vi "Test Test Pass if Expected API Call Made Asynchronously.vi"(8 "error in (no error)":errorcluster, 11 "Test Case In":refnum<class "One Expectation Test.lvclass">) -> (0 "error out":errorcluster, 3 "Test Case Out":refnum<class "One Expectation Test.lvclass">)   [LabVIEW 2020, in "One Expectation Test.lvclass"]
uses:
  One Expectation Test.lvclass
  C:/Program Files (x86)/National Instruments/LabVIEW 2020/vi.lib/Astemes/LUnit/Test Case.lvclass
  <vilib>/Astemes/LUnit/Test Case.lvclass
  <vilib>/Astemes/LUnit/Test Case.lvclass/Test Case.ctl
  6053ebfb-fa78-43cc-b4be-896e65d0506d.vi
  <vilib>/Astemes/LUnit/Append Pass Result.vi
  <vilib>/Astemes/LUnit/Append Fail Result.vi
  <vilib>/Astemes/LUnit/Describe Comparison.vi
  <vilib>/Astemes/LUnit/Compare Variants.vi
  <vilib>/Astemes/LUnit/Variant to string.vi
  Test Interface Mock/Test Interface Mock.lvclass
  C:/git/astemes-lmock/sandbox/Mock/Mock.lvclass
  <vilib>/Utility/Data Type/Get Type Information.vi
  <vilib>/Utility/LVClass/Get LV Class Name.vi
  One Of/One.lvclass
  Validator/Verifier.lvclass
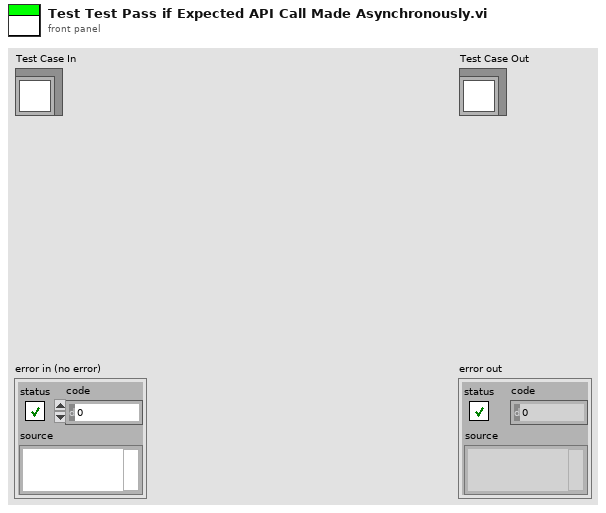
[diagram p1: front panel]
types:
  T1 = enum16{"", "Passed", "Failed", "Error", "Skipped", "Setup Error", "Broken", "Teardown Error"}
  T2 = cluster{"Name":string, "Message":string, "Description":string, "Status":enum16{"", "Passed", "Failed", "Error", "Skipped", "Setup Error", "Broken", "Teardown Error"}, "Result Type":enum16{"Test Case", "Test Suite", "Test Run", "Pass", "Fail", "Skip", "Pass if", "Fail if", "Pass if Error", "Fail if Error", "Pass if Equal", "Fail if Equal"}, "Execution Time":dbl}[]
  T3 = cluster{"Name":string, "Message":string, "Description":string, "Status":enum16{"", "Passed", "Failed", "Error", "Skipped", "Setup Error", "Broken", "Teardown Error"}, "Result Type":enum16{"Test Case", "Test Suite", "Test Run", "Pass", "Fail", "Skip", "Pass if", "Fail if", "Pass if Error", "Fail if Error", "Pass if Equal", "Fail if Equal"}, "Execution Time":dbl}
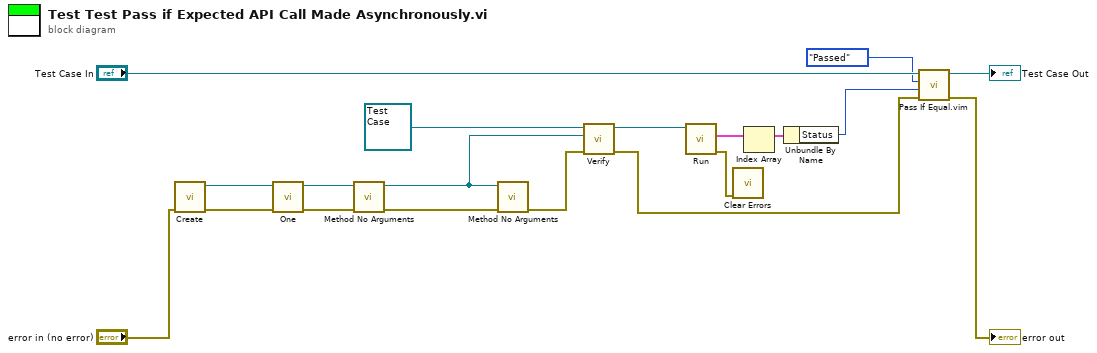
[diagram p0: block diagram]
diagram:
  n1 = call "Create.vi"("error in (no error)"="error in (no error)") -> ("error out"=w18:errorcluster, "Test Interface Mock Out"=w19:refnum<class "Test Interface Mock.lvclass">)  [unwired: 9 in]
  n2 = call "One.vi"("error in (no error)"=w18, "Mock in"=w19) -> ("error out"=w16:errorcluster, "Mock out"=w17:refnum<class "Test Interface Mock.lvclass">)  [unwired: 8 in]
  n3 = call-dynamic "Method No Arguments.vi"("error in (no error)"=w16, "Mock In"=w17) -> ("error out"=w15:errorcluster, "Mock Out"=w1:refnum<class "Test Interface Mock.lvclass">)  [unwired: 8 in]
  n4 = call-dynamic "Method No Arguments.vi"("error in (no error)"=w15, "Mock In"=w1) -> ("error out"=w2:errorcluster)  [unwired: 8 in, 1 out]
  n5 = call "Verify.vi"("error in (no error)"=w2, "Mock.lvclass"=w1, "LUnit Test Case In"=refnum<class "Test Case.lvclass"> refnum) -> ("error out"=w14:errorcluster, "LUnit Test Case Out"=w8:refnum<class "Test Case.lvclass">)  [unwired: 7 in]
  n6 = call-dynamic "Run.vi"("LUnit Test Case In"=w8) -> ("error out"=w3:errorcluster, "Results"=w7:T2)  [unwired: 7 in, 2 out]
  n7 = call <vilib>:"Clear Errors.vi"("error in (no error)"=w3) -> ()  [unwired: 5 in, 2 out]
  n8 = Index Array(array=w7) -> (element=w6:T3)  [unwired: 1 in]
  n9 = Unbundle By Name(w6) -> ("Status"=w5:T1)
  n10 = call "Pass If Equal.vim"("error in (no error)"=w14, "Actual"=w5, "Expected"=T1."Passed" ("Status"), "LUnit Test Case In"="Test Case In") -> ("error out"=→"error out":errorcluster, "LUnit Test Case Out"=→"Test Case Out":refnum<class "One Expectation Test.lvclass">)  [unwired: 6 in]
